vi "LAB2_LABVIEW.vi"() -> ()   [LabVIEW 2025]
panel:
  out "Boolean":bool
  out "Flow Rate L/min":dbl(slide) scale=-40000.0..40000.0 scale format="%#8.0g"
  out "Sensor,V":dbl
  out "SCC,V":dbl
  out "AtoD":i16 format="%x"
  in  "stop":bool
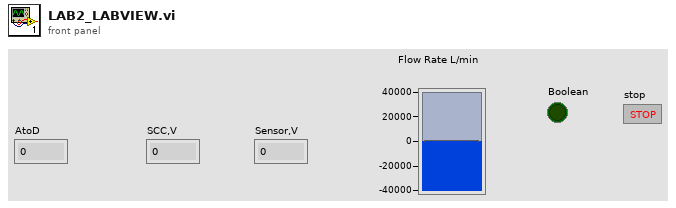
[diagram p1: front panel]
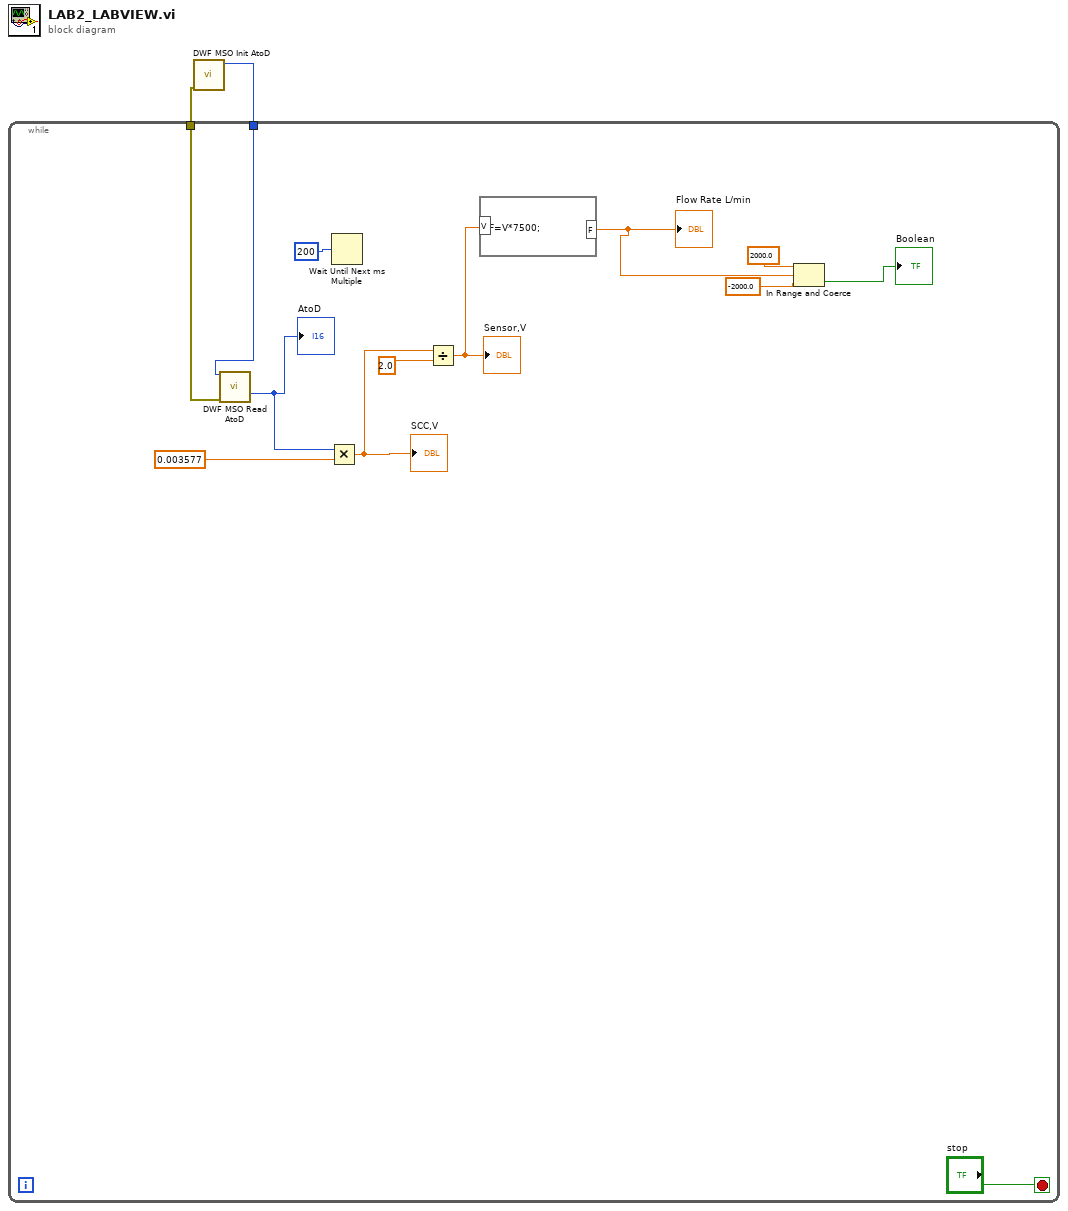
[diagram p0: block diagram]
diagram:
  n1 = call "DWF MSO Init AtoD.vi"() -> ("Error Out"=w1:errorcluster, "Instrument Handle Out"=w2:i32)  [unwired: 10 in]
  n2 = while {
    tunnel: w2 -> [w14]
    tunnel: w1 -> [w13]
    stop <- "stop" stop-if-true
    n3 = call "DWF MSO Read AtoD.vi"("Instrument Handle In AtoD"=w14, "Error In"=w13) -> ("AtoD"=w11:i16)  [unwired: 12 in, 1 out]
    "AtoD" <- w11
    n4 = Multiply(x=w11, y=0.003577) -> (x*y=w8:dbl)
    "SCC,V" <- w8
    n5 = Wait Until Next ms Multiple(millisecond multiple=u32 200) -> ()  [unwired: 1 out]
    n6 = Divide(x=w8, y=2.0) -> (x/y=w7:dbl)
    "Sensor,V" <- w7
    n7 = formula code="F=V*7500;"("V"=w7) -> ("F"=w4:dbl)
    "Flow Rate L/min" <- w4
    n8 = In Range and Coerce(upper limit=2000.0, x=w4, lower limit=-2000.0) -> (In Range?=→"Boolean":bool)  [unwired: 1 out]
  }
